vi "Compile Settings.vi"(8 "error in":errorcluster, 10 "Settings(JSON)":string, 11 "Custom Device Deployment Hooks in":refnum<class "Custom Device Deployment Hooks.lvclass">) -> (0 "error out":errorcluster, 2 "Compiled Settings":variant, 3 "Custom Device Deployment Hooks out":refnum<class "Custom Device Deployment Hooks.lvclass">)   [LabVIEW 2027, in "Custom Device Interfaces.lvlib" / "Custom Device Deployment Hooks.lvclass"]
uses:
  Custom Device Deployment Hooks.lvclass
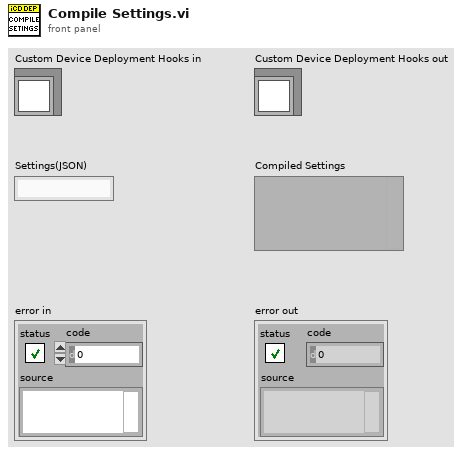
[diagram p1: front panel]
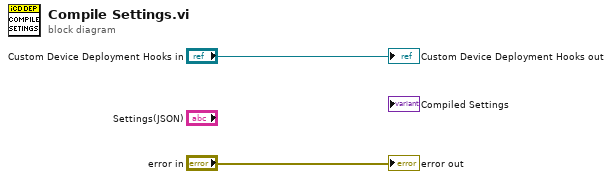
[diagram p0: block diagram]
diagram:
  "error out" <- "error in"
  "Custom Device Deployment Hooks out" <- "Custom Device Deployment Hooks in"
